vi "未命名 4.vi"(0 "输入":dbl) -> (1 "正弦":dbl, 2 "余弦":dbl)   [LabVIEW 2017]
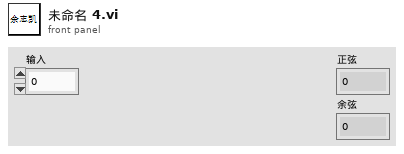
[diagram p1: front panel]
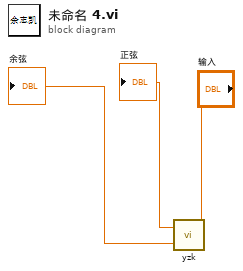
[diagram p0: block diagram]
diagram:
  n1 = call "yzk.vi"("输入"="输入") -> ("余弦"=→"余弦":dbl, "正弦"=→"正弦":dbl)
